vi "SeCrTs-Drive_Read_A.vi"(8 "error in":errorcluster, 9 "Er":refnum<queue>, 11 "Data FIFO Ref":T1) -> (0 "error out":errorcluster)   [LabVIEW 2022 SP3]
uses:
  Pumb PXie/RT Support/SeCrTs-RT_Global_R.vi
  RT Controls/ATF Storage-Data FIFO.ctl
panel:
  in  "TCP_Port_Bottom":u16=3000
  in  "TCP_Port_Top":u16=2000
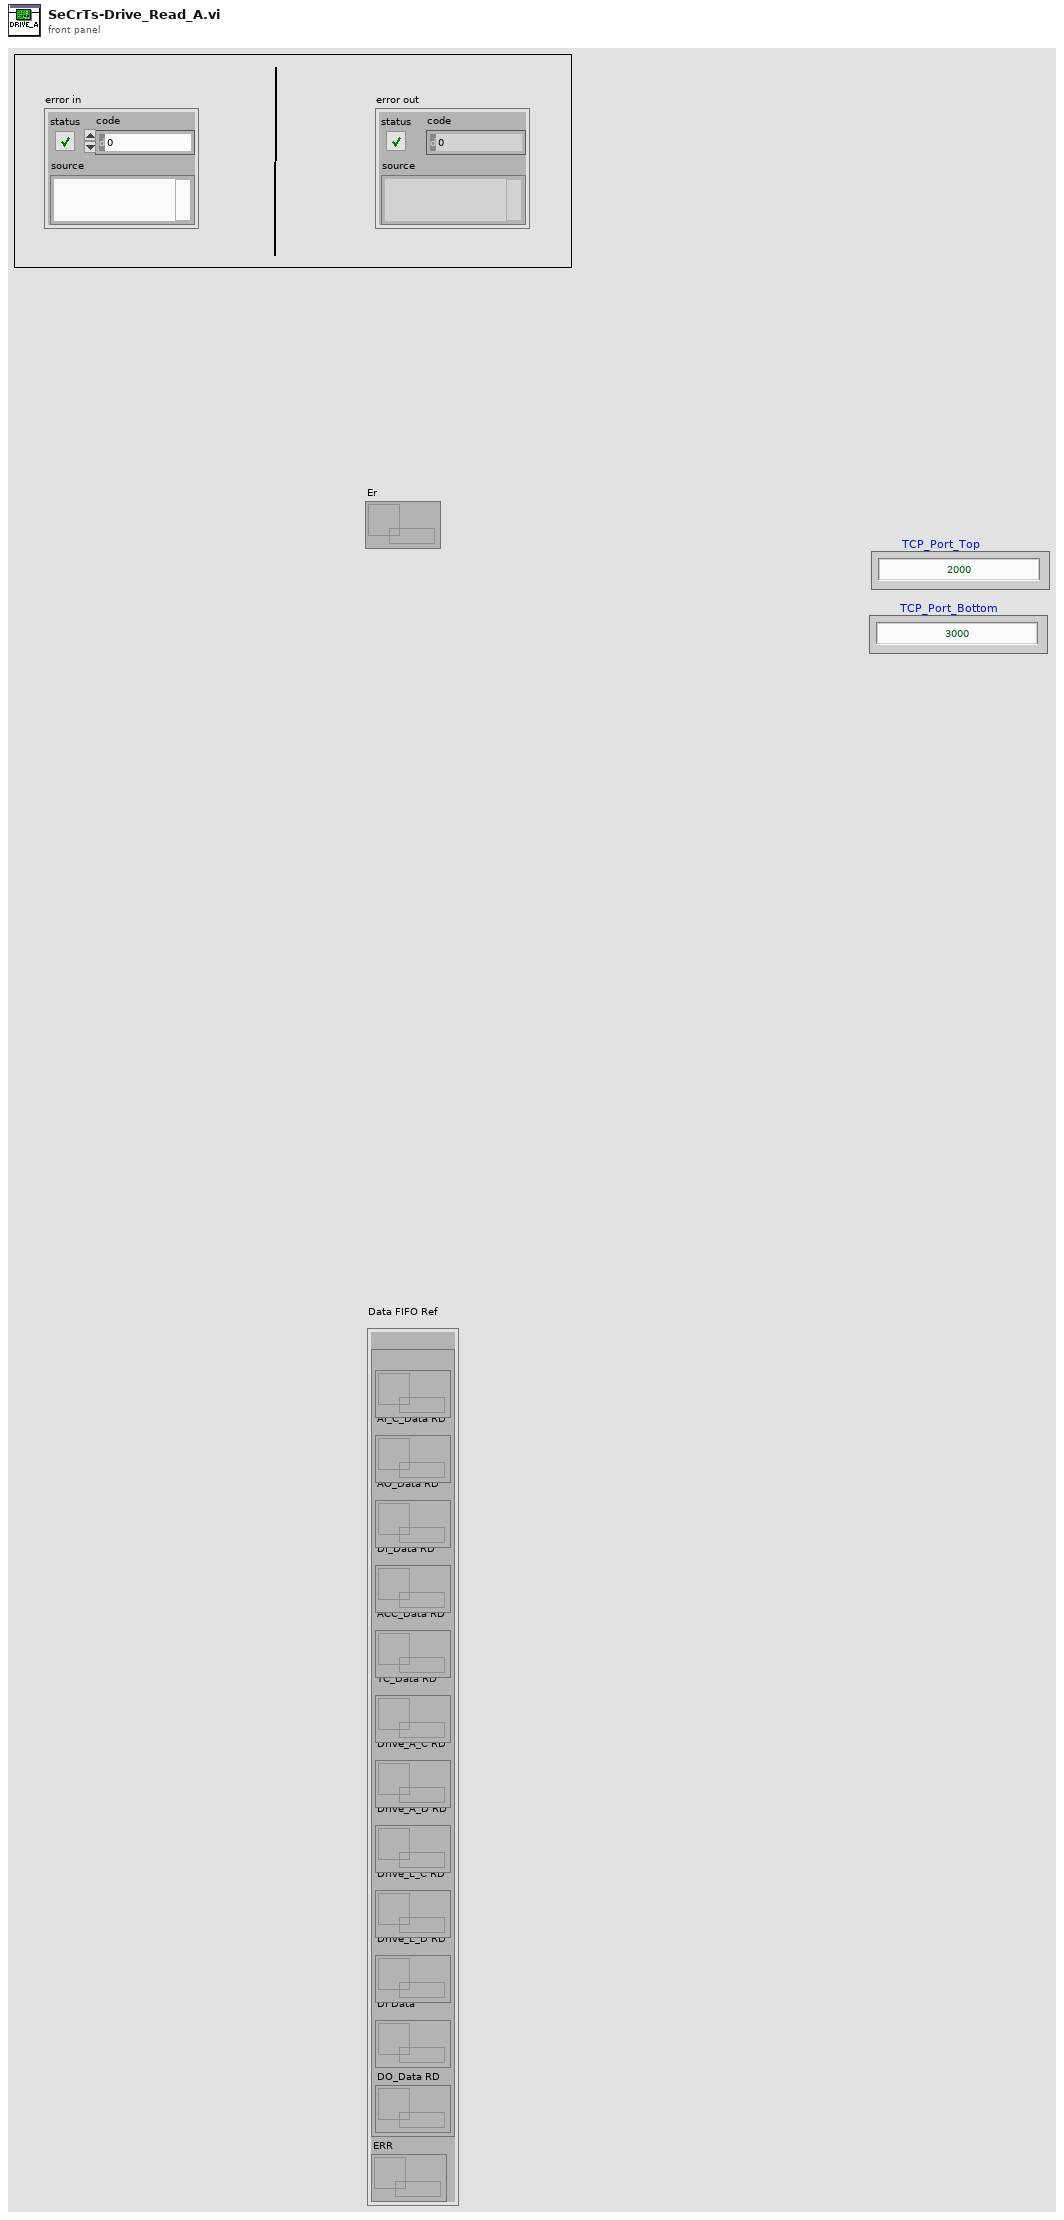
[diagram p1: front panel]
types:
  T1 = typedef "ATF Storage-Data FIFO.ctl" = cluster{"RD":cluster{"AI_V_Data RD":refnum<queue>, "AI_C_Data RD":refnum<queue>, "AO_Data RD":refnum<queue>, "DI_Data RD":refnum<queue>, "ACC_Data RD":refnum<queue>, "TC_Data RD":refnum<queue>, "Drive_A_C RD":refnum<queue>, "Drive_A_D RD":refnum<queue>, "Drive_L_C RD":refnum<queue>, "Drive_L_D RD":refnum<queue>, "DI Data":refnum<queue>, "DO_Data RD":refnum<queue>}, "ERR":refnum<queue>}
  T2 = enum16{"AI C", "AI V", "AO", "DI", "DO", "TC", "ACC", "DR L", "DR A"}
  T3 = enum16{"Init", "Read 'All'", "Read 'n'", "Read '1'", "Write '1'", "Write 'n'", "Write 'All'"}
  T4 = cluster{"Start DAQ":bool, "Stop DAQ":bool, "RT Stop":bool, "RT Exit":bool, "Start Seq":bool}
  T5 = cluster{"En_Drive_A":bool, "En_Drive_L":bool, "Exit_Drive_A":bool, "Exit_Drive_L":bool}
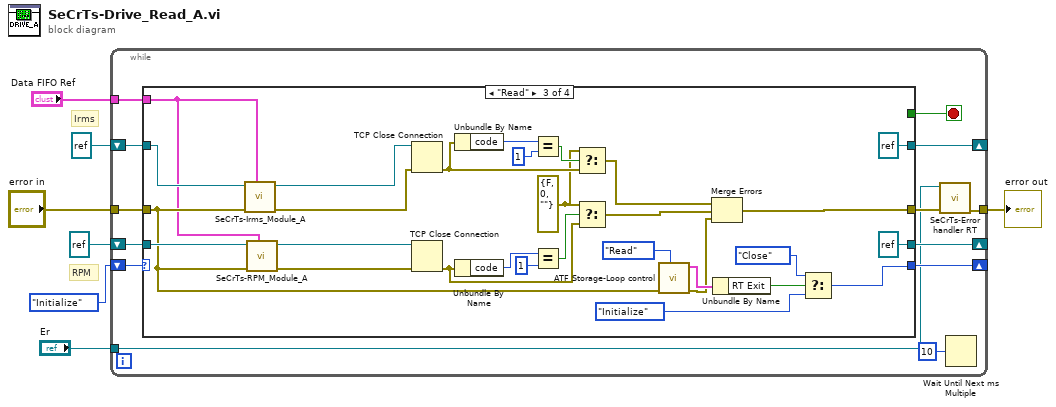
[diagram p0: block diagram]
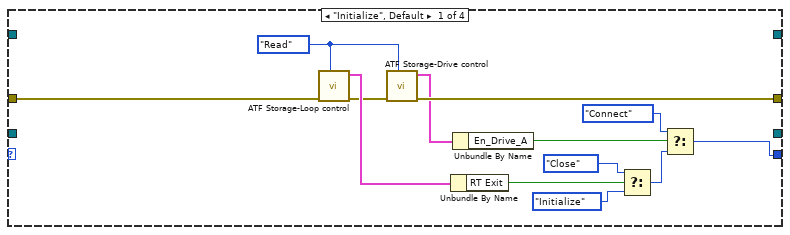
[diagram p2: hidden frame]
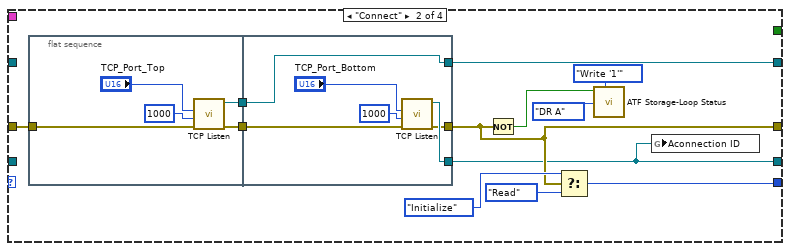
[diagram p3: hidden frame]
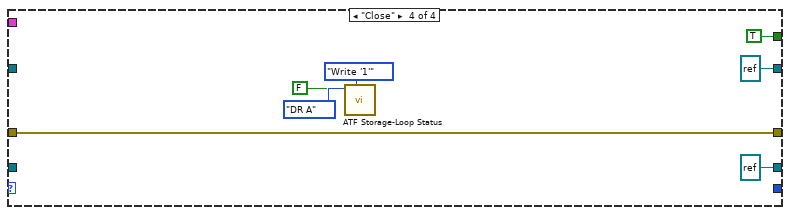
[diagram p4: hidden frame]
diagram:
  # "RPM"
  # "Irms"
  n1 = while {
    shift-right: [w19] -> _
    shift-left: enum16{"Initialize", "Connect", "Read", "Close"}."Initialize" -> [w20]
    tunnel: "error in" -> [w18]
    tunnel: [w10] -> w5
    shift-right: [w17] -> _
    shift-left: refnum<k5> refnum ("connection ID") -> [w15]
    shift-right: [w16] -> _
    shift-left: refnum<k5> refnum ("connection ID") -> [w14]
    tunnel: "Data FIFO Ref" -> [w12]
    tunnel: "Er" -> [w9]
    stop <- w13 stop-if-true
    n2 = case shown="\"Read\"" w20 {
      tunnel: [w33 w39 w83 _] -> w19
      tunnel: w18 -> [w26 w43 w58 w89]
      tunnel: [w25 w38 w71 w89] -> w11
      tunnel: [_ w42 refnum<k5> refnum ("TCP Network Connection out") refnum<k5> refnum ("TCP Network Connection out")] -> w17
      tunnel: [_ w37 refnum<k5> refnum ("TCP Network Connection out") refnum<k5> refnum ("TCP Network Connection out")] -> w16
      tunnel: w15 -> [_ _ w66 _]
      tunnel: w14 -> [_ _ w65 _]
      tunnel: [_ _ _ TRUE] -> w13
      tunnel: w12 -> [_ _ w57 _]
      frame "Initialize", Default {
        w21 = enum16{"Init", "Write", "Read"}."Read" ("Action")
        n3 = call "ATF Storage-Loop control.vi"("Action"=w21, "error in (no error)"=w26) -> ("error Out"=w24:errorcluster, "Loop Control out"=w28:T4)  [unwired: 8 in]
        n4 = call "ATF Storage-Drive control.vi"("Action"=w21, "error in"=w24) -> ("error Out"=w25:errorcluster, "Loop Control Out"=w23:T5)  [unwired: 8 in]
        n5 = Unbundle By Name(w28) -> ("RT Exit"=w27:bool)
        n6 = Unbundle By Name(w23) -> ("En_Drive_A"=w22:bool)
        n7 = Select(t=enum16{"Initialize", "Connect", "Read", "Close"}."Close", s=w27, f=enum16{"Initialize", "Connect", "Read", "Close"}."Initialize") -> (s? t:f=w29:enum16{"Initialize", "Connect", "Read", "Close"})
        n8 = Select(t=enum16{"Initialize", "Connect", "Read", "Close"}."Connect", s=w22, f=w29) -> (s? t:f=w33:enum16{"Initialize", "Connect", "Read", "Close"})
      }
      frame "Connect" {
        n9 = flat-sequence {
          tunnel: w43 -> [w48]
          tunnel: [w47] -> w45
          tunnel: [w46] -> w44
          tunnel: [w56] -> w37
          tunnel: w45 -> [w52]
          tunnel: w44 -> [w55]
          tunnel: [w55] -> w42
          tunnel: [w51] -> w38
          frame #0 {
            n10 = call <vilib>:"TCP Listen.vi"("error in (no error)"=w48, "timeout ms (wait forever: -1)"=1000, "port"="TCP_Port_Top") -> ("error out"=w47:errorcluster, "connection ID"=w46:refnum<k5>)  [unwired: 4 in, 3 out]
          }
          frame #1 {
            n11 = call <vilib>:"TCP Listen.vi"("error in (no error)"=w52, "timeout ms (wait forever: -1)"=1000, "port"="TCP_Port_Bottom") -> ("error out"=w51:errorcluster, "connection ID"=w56:refnum<k5>)  [unwired: 4 in, 3 out]
          }
        }
        n12 = Not(x=w38) -> (.not. x?=w34:bool)
        n13 = Select(t=enum16{"Initialize", "Connect", "Read", "Close"}."Initialize", s=w38, f=enum16{"Initialize", "Connect", "Read", "Close"}."Read") -> (s? t:f=w39:enum16{"Initialize", "Connect", "Read", "Close"})
        n14 = call "ATF Storage-Loop Status.vi"("Option"=T3."Write '1'", "Status"=w34, "Loop"=T2."DR A") -> ()  [unwired: 6 in, 3 out]
        n15 = global write "SeCrTs-RT_Global_R.vi" "Aconnection ID"(w37) -> ()
      }
      frame "Read" {
        w74 = errorcluster {"status"=FALSE, "code"=0, "source"=""} ("error constant")
        n16 = call "SeCrTs-Irms_Module_A.vi"("Data FIFO Ref"=w57, "error in"=w58, "TCP Network Connection in"=w66) -> ("error out"=w67:errorcluster, "TCP Network Connection out"=w68:refnum<k5>)  [unwired: 7 in]
        n17 = call "SeCrTs-RPM_Module_A.vi"("Data FIFO Ref"=w57, "error in (no error)"=w58, "TCP Network Connection in"=w65) -> ("error out"=w63:errorcluster, "TCP Network Connection out"=w64:refnum<k5>)  [unwired: 7 in]
        n18 = TCP Close Connection(connection ID=w68, error in (no error)=w67) -> (error out=w78:errorcluster)  [unwired: 1 in, 1 out]
        n19 = TCP Close Connection(connection ID=w64, error in (no error)=w63) -> (error out=w77:errorcluster)  [unwired: 1 in, 1 out]
        n20 = Unbundle By Name(w78) -> ("code"=w82:i32)
        n21 = Unbundle By Name(w77) -> ("code"=w81:i32)
        n22 = Equal?(x=w82, y=1) -> (x = y?=w79:bool)
        n23 = Equal?(x=w81, y=1) -> (x = y?=w80:bool)
        n24 = Select(t=w74, s=w79, f=w78) -> (s? t:f=w76:errorcluster)
        n25 = Select(t=w74, s=w80, f=w77) -> (s? t:f=w75:errorcluster)
        n26 = call "ATF Storage-Loop control.vi"("Action"=enum16{"Init", "Write", "Read"}."Read", "error in (no error)"=w58) -> ("error Out"=w59:errorcluster, "Loop Control out"=w62:T4)  [unwired: 8 in]
        n27 = Merge Errors(w76, w75, w59) -> (w71:errorcluster)
        n28 = Unbundle By Name(w62) -> ("RT Exit"=w61:bool)
        n29 = Select(t=enum16{"Initialize", "Connect", "Read", "Close"}."Close", s=w61, f=enum16{"Initialize", "Connect", "Read", "Close"}."Initialize") -> (s? t:f=w83:enum16{"Initialize", "Connect", "Read", "Close"})
      }
      frame "Close" {
        n30 = call "ATF Storage-Loop Status.vi"("Option"=T3."Write '1'", "Status"=FALSE, "Loop"=T2."DR A") -> ()  [unwired: 6 in, 3 out]
      }
    }
    n31 = call "SeCrTs-Error handler RT.vi"("error in"=w11, "Message Queue"=w9) -> ("error out"=w10:errorcluster)  [unwired: 8 in, 1 out]
    n32 = Wait Until Next ms Multiple(millisecond multiple=u32 10) -> ()  [unwired: 1 out]
  }
  "error out" <- w5
